vi "Create Headless.vi"(8 "error in":errorcluster, 9 "Resolution":i32) -> (0 "error out":errorcluster, 3 "BigMAQ out":refnum<class "BigMAQ.lvclass">)   [LabVIEW 2019, in "BigMAQ.lvclass"]
uses:
  BigMAQ.lvclass
  BigMAQ.lvclass/BigMAQ.ctl
panel:
  in  "BigMAQ in":refnum<class "BigMAQ.lvclass">
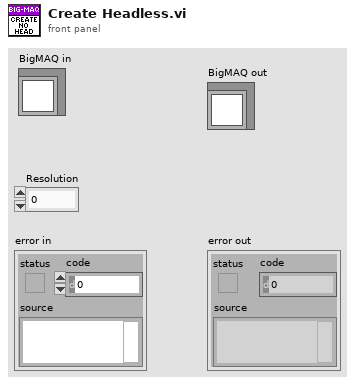
[diagram p1: front panel]
types:
  T1 = typedef "IMAQ Image.ctl" = refnum<image>
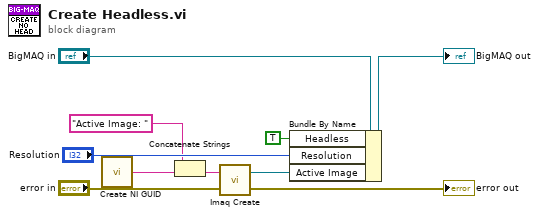
[diagram p0: block diagram]
diagram:
  n1 = call "Create NI GUID.vi"() -> ("NI GUID"=w1:string)
  n2 = Concatenate Strings("Active Image: " ("Image Name"), w1) -> (w5:string)
  n3 = call "Imaq Create"("Image Name"=w5, "error in (no error)"="error in") -> ("New Image"=w3:T1, "error out"=→"error out":errorcluster)  [unwired: 3 in]
  n4 = Bundle By Name(cluster="BigMAQ in", "Headless"=TRUE, "Resolution"="Resolution", "Active Image"=w3) -> (→"BigMAQ out":refnum<class "BigMAQ.lvclass">)
